vi "BGCorrection.vi"(2 "Boolean":bool, 3 "channels":u8[](array[numeric])=[1, 2, 3], 4 "MCS":u32[][](array[numeric])) -> (0 "BG_mcs":sgl[](array[numeric]) format="%.2f", 1 "MCS_bg_corr":sgl[][](array[numeric]) format="%.2f")   [LabVIEW 2009]
uses:
  <vilib>/Analysis/NI_AALPro.lvlib
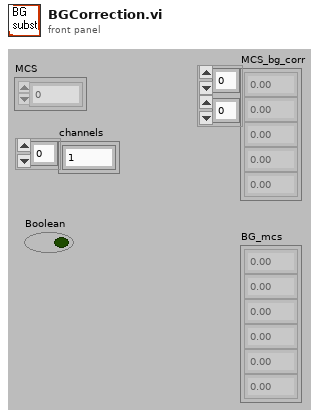
[diagram p1: front panel]
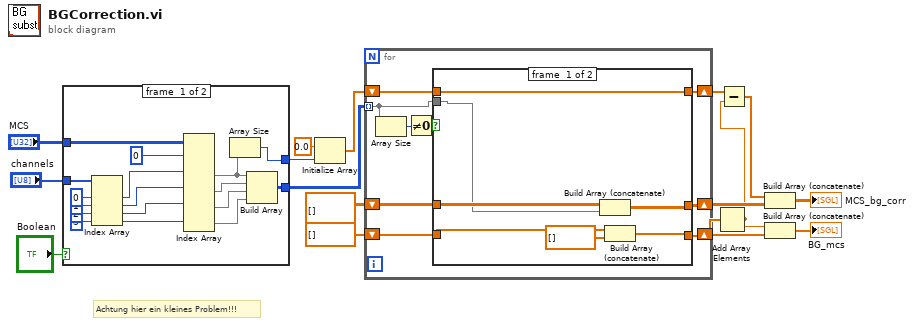
[diagram p0: block diagram]
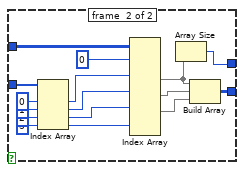
[diagram p2: hidden frame]
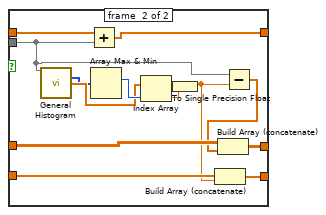
[diagram p3: hidden frame]
diagram:
  # "Achtung hier ein kleines Problem!!!"
  n1 = case shown="True" "Boolean" {
    tunnel: "MCS" -> [w33 w49]
    tunnel: "channels" -> [w25 w41]
    tunnel: [w19 w35] -> w11
    tunnel: [w18 w34] -> w5
    frame #0 {
      n2 = Index Array(array=w25, index #1=0 ("index"), index #2=1 ("index"), index #3=2 ("index"), index #4=3 ("index")) -> (element #1=w21:u8, element #2=w22:u8, element #3=w23:u8, element #4=w24:u8)
      n3 = Index Array(array=w33, index (row) #1=0 ("index (row)"), index (row) #2=w21, index (row) #3=w22, index (row) #4=w23, index (row) #5=w24) -> (element #2=w20:u32[], element #3=w31:u32[], element #4=w30:u32[], element #5=w17:u32[])  [unwired: 5 in, 1 out]
      n4 = Array Size(array=w20) -> (size(s)=w18:i32)
      n5 = Build Array(w20, w31, w30, w17) -> (w19:u32[][])
    }
    frame #1 {
      n6 = Index Array(array=w41, index #1=0 ("index"), index #2=1 ("index"), index #3=2 ("index"), index #4=3 ("index")) -> (element #1=w37:u8, element #2=w38:u8, element #3=w39:u8, element #4=w40:u8)
      n7 = Index Array(array=w49, index (row) #1=0 ("index (row)"), index (row) #2=w37, index (row) #3=w38, index (row) #4=w39, index (row) #5=w40) -> (element #2=w36:u32[], element #3=w47:u32[], element #4=w46:u32[])  [unwired: 5 in, 2 out]
      n8 = Array Size(array=w36) -> (size(s)=w34:i32)
      n9 = Build Array(w36, w47, w46) -> (w35:u32[][])
    }
  }
  n10 = Initialize Array(sgl 0.0 ("element"), w5) -> (w6:sgl[])
  n11 = for {
    tunnel: w11 -> [w54] mode=indexing
    shift-right: [w57] -> w13
    shift-left: w6 -> [w56]
    shift-right: [w50] -> w8
    shift-left: sgl[][] [] -> [w53]
    shift-right: [w51] -> w7
    shift-left: sgl[] [] -> [w52]
    n12 = Array Size(array=w54) -> (size(s)=w55:i32)
    n13 = Not Equal To 0?(x=w55) -> (x != 0?=w58:bool)
    n14 = case shown="False" w58 {
      tunnel: w54 -> [w62 w72]
      tunnel: [w65 w77] -> w57
      tunnel: w56 -> [w65 w78]
      tunnel: [w63 w71] -> w50
      tunnel: w53 -> [w64 w70]
      tunnel: w52 -> [w61 w68]
      tunnel: [w60 w67] -> w51
      frame #0 {
        n15 = Build Array (concatenate)(w64, w62) -> (w63:sgl[][])
        n16 = Build Array (concatenate)(w61, sgl[] [] ("array")) -> (w60:sgl[])
      }
      frame #1 {
        n17 = call <vilib>:"General Histogram.vi"("X"=w72) -> ("Histogram"=w73:i32[], "Axis"=w74:dbl[])  [unwired: 10 in, 3 out]
        n18 = Add(x=w78, y=w72) -> (x+y=w77:sgl[])
        n19 = Array Max & Min(array=w73) -> (max index (indices)=w75:i32)  [unwired: 3 out]
        n20 = Index Array(array=w74, index=w75) -> (element=w76:dbl)
        n21 = To Single Precision Float(number=w76) -> (single precision float=w66:sgl)
        n22 = Build Array (concatenate)(w68, w66) -> (w67:sgl[])
        n23 = Subtract(x=w72, y=w66) -> (x-y=w69:sgl[])
        n24 = Build Array (concatenate)(w70, w69) -> (w71:sgl[][])
      }
    }
  }
  n25 = Add Array Elements(numeric array=w7) -> (sum=w2:sgl)
  n26 = Subtract(x=w13, y=w2) -> (x-y=w10:sgl[])
  n27 = Build Array (concatenate)(w10, w8) -> (→"MCS_bg_corr":sgl[][])
  n28 = Build Array (concatenate)(w2, w7) -> (→"BG_mcs":sgl[])
